vi "WPI_SerialPortClose.vi"(8 "error in (no error)":errorcluster, 11 "SerialPortRef":T1) -> (0 "error out":errorcluster)   [LabVIEW 2017]
doc: "Closes the reference to the serial port you specify. Use this VI to close each serial port reference that you open with the Open VI.\n\nThis software is licensed. Open the labview\\readme\\WPI Robotics Library Open Source License.txt file for more information."
uses:
  <vilib>/Rock Robotics/WPI/SerialPort/WPI_SerialPortRef.ctl
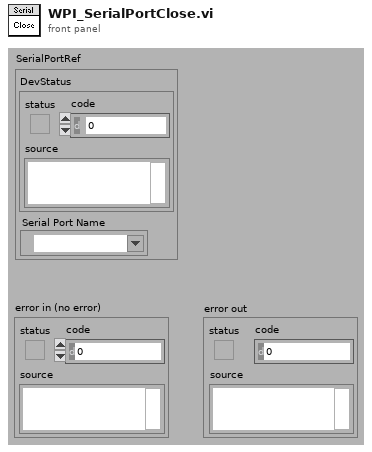
[diagram p1: front panel]
types:
  T1 = typedef "WPI_SerialPortRef.ctl" = cluster{"DevStatus":errorcluster, "Serial Port Name":refnum<visa-resource-name>}
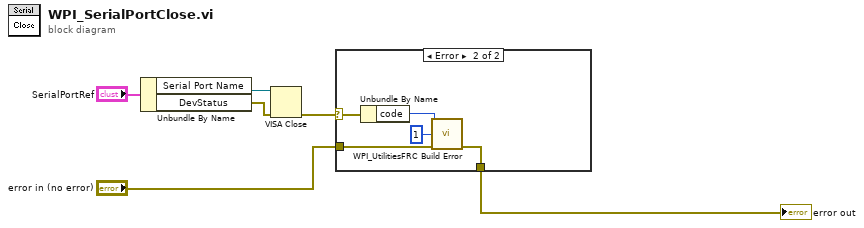
[diagram p0: block diagram]
diagram:
  n1 = Unbundle By Name("SerialPortRef") -> ("Serial Port Name"=w5:refnum<visa-resource-name>, "DevStatus"=w4:errorcluster)
  n2 = VISA Close(VISA resource name=w5, error in (no error)=w4) -> (error out=w3:errorcluster)
  n3 = case shown="Error" w3 {
    selector: w3 -> [w7 w11]
    tunnel: [w7 w9] -> w1
    tunnel: "error in (no error)" -> [_ w8]
    frame No Error {
    }
    frame Error {
      n4 = Unbundle By Name(w11) -> ("code"=w10:i32)
      n5 = call <vilib>:"WPI_UtilitiesFRC Build Error.vi"("error code"=w10, "chain levels to remove (1)"=1, "error in (no error)"=w8) -> ("error out"=w9:errorcluster)  [unwired: 2 in, 10 out]
    }
  }
  "error out" <- w1
